vi "IOclocktest.vi"() -> ()   [LabVIEW 2012]
uses:
  <vilib>/platform/TimedLoop/XDataNode/XDataNode.xnode
  <vilib>/Platform/TimedLoop/XDataNode/nitl_modes.ctl
  <vilib>/Platform/TimedLoop/XDataNode/XDNodeRunTimeDep.lvlib
  <vilib>/Platform/TimedLoop/XDataNode/wakeup.ctl
  <vilib>/Platform/TimedLoop/XDataNode/timing_clust.ctl
  <vilib>/eio/EIONode/EIONode.xnode
  <vilib>/rvi/eio/common/nirviEmuTemplateMethod_errors.vi
panel:
  out "Numeric 2":i32
  out ".not. x? 2":bool
  out ".not. x?":bool
  out "Numeric":i32
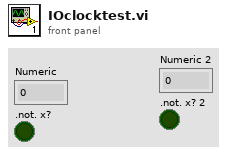
[diagram p1: front panel]
types:
  T1 = typedef "XDNodeRunTimeDep.lvlib/timing_clust.ctl" = cluster{"Expected End [f-1]":u64, "Actual End [f-1]":u64, "Finished Late? [f-1]":bool, "Expected End [i-1]":u64, "Actual End [i-1]":u64, "Finished Late? [i-1]":bool, "Expected Start [i]":u64, "Actual Start [i]":u64, "Expected Start [f]":u64, "Actual Start [f]":u64, "Source Name":string, "Structure Name":string, "Period":i64, "Deadline":i64, "Offset":i64, "Start":i64, "Priority":i32, "Timeout":i32, "Mode":T2, "Wakeup Reason":T3, "Error":errorcluster, "Source Type":string, "Secondary Source Type":string, "Global End Time":u64, "Global Start Time":u64, "Frame Duration":u64, "Iteration Duration":u64, "Assigned CPU":i32, "I/O Scan Engine Mode":u32}
  T2 = typedef "XDNodeRunTimeDep.lvlib/nitl_modes.ctl" = enum32{"No Change", "Process missed periods, maintain original phase", "Discard missed periods, maintain original phase", "Process missed periods, ignore original phase", "Discard missed periods, ignore original phase"}
  T3 = typedef "XDNodeRunTimeDep.lvlib/wakeup.ctl" = enum32{"Normal", "Aborted", "Asynchronous wakeup", "Timing source error", "Timed loop error", "Timeout"}
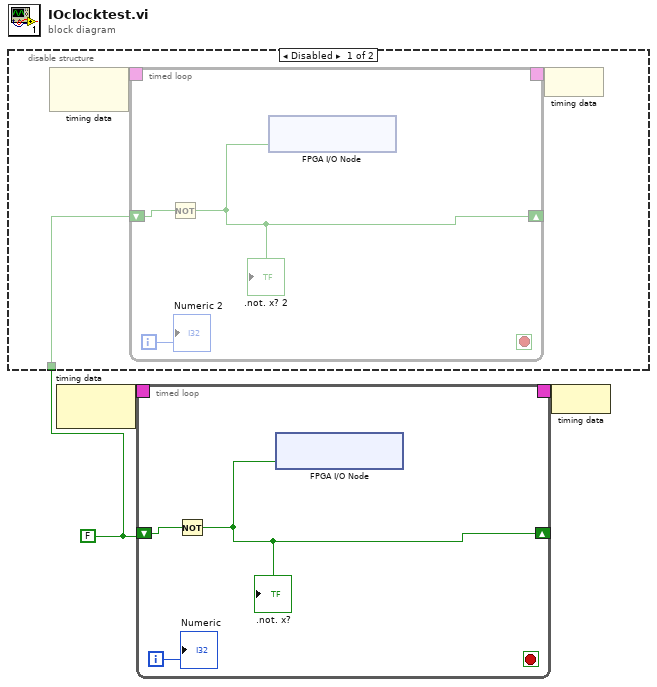
[diagram p0: block diagram]
diagram:
  w1 = FALSE ("IO Module\\D0 0")
  n1 = disable-structure shown="Disabled" {
    disable-tunnel: w1 -> [w4 _]
    frame Disabled {
      n2 = node-c288() -> (w6:T1)  [unwired: 1 in]
      n3 = timed-loop {
        timing: w6 -> [_]
        timing-out: [_] -> w5
        shift-right: [w8] -> _
        shift-left: w4 -> [w9]
        i -> [w7]
        stop <- _ stop-if-true
        n4 = Not(x=w9) -> (.not. x?=w8:bool)
        ".not. x? 2" <- w8
        n5 = xnode "FPGA I/O Node"("IO Module\\D0 1"=w8) -> ()  [unwired: 1 in, 1 out]
        "Numeric 2" <- w7
      }
      n6 = node-c288(w5) -> ()
    }
    frame Enabled {
    }
  }
  n7 = node-c288() -> (w3:T1)  [unwired: 1 in]
  n8 = timed-loop {
    timing: w3 -> [_]
    timing-out: [_] -> w2
    shift-right: [w15] -> _
    shift-left: w1 -> [w16]
    i -> [w14]
    stop <- _ stop-if-true
    n9 = Not(x=w16) -> (.not. x?=w15:bool)
    ".not. x?" <- w15
    n10 = xnode "FPGA I/O Node"("IO Module\\D0 0"=w15) -> ()  [unwired: 1 in, 1 out]
    "Numeric" <- w14
  }
  n11 = node-c288(w2) -> ()
